vi "TL_convert_cluster into_TDMS_array.vi"(2 "TL cluster":T2={"405"=0.0, "488"=0.0, "561"=0.0, "641"=0.0, "BF "=0.0, "405 setpoint"=FALSE, "488 setpoint"=FALSE, "561 setpoint"=FALSE, "641 setpoint"=FALSE, "BF setpoint"=FALSE, "N planes 405"=0, "Dz 405"=0, "N planes 488"=0, "Dz 488"=0, "N planes 561"=0, "Dz 561"=0, "N planes 641"=0, "Dz 641"=0, "N planes BF"=0, "Dz BF"=0, "Tau 405"=inf, "Tau 488"=inf, "Tau 561"=inf, "Tau 641"=inf, "Tau BF"=inf, "405 set"=FALSE, "488 set "=FALSE, "561 set"=FALSE, "641 set"=FALSE, "BF set"=FALSE} {"Tau BF" format="%#_6e"; "Tau 641" format="%#_6e"; "Tau 561" format="%#_6e"; "Tau 488" format="%#_6e"; "Tau 405" format="%#_6e"; "641" min=0.0 max=100.0 step=0.1 scale=0.0..100.0; "561" min=0.0 max=100.0 step=0.1 scale=0.0..100.0; "405" min=0.0 max=100.0 step=0.1 scale=0.0..100.0; "488" min=0.0 max=100.0 step=0.1 scale=0.0..100.0; "BF" min=0.0 max=100.0 step=0.1 scale=0.0..100.0}, 3 "TL - setpoint cluster":T1) -> (0 "TL data for TDMS":cluster{dbl[][], dbl[][]})   [LabVIEW 2015]
uses:
  CONTROLS/Time_lapse_parameters.ctl
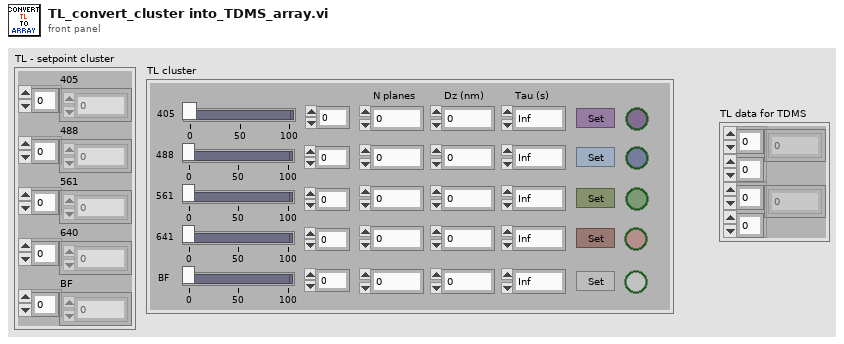
[diagram p1: front panel]
types:
  T1 = cluster{"405":dbl[], "488":dbl[], "561":dbl[], "640":dbl[], "BF":dbl[]}
  T2 = typedef "Time_lapse_parameters.ctl" = cluster{"405":dbl, "488":dbl, "561":dbl, "641":dbl, "BF ":dbl, "405 setpoint":bool, "488 setpoint":bool, "561 setpoint":bool, "641 setpoint":bool, "BF setpoint":bool, "N planes 405":i32, "Dz 405":i32, "N planes 488":i32, "Dz 488":i32, "N planes 561":i32, "Dz 561":i32, "N planes 641":i32, "Dz 641":i32, "N planes BF":i32, "Dz BF":i32, "Tau 405":dbl, "Tau 488":dbl, "Tau 561":dbl, "Tau 641":dbl, "Tau BF":dbl, "405 set":bool, "488 set ":bool, "561 set":bool, "641 set":bool, "BF set":bool}
  T3 = cluster{"Setpoint":dbl[][], "parameters":dbl[][]}
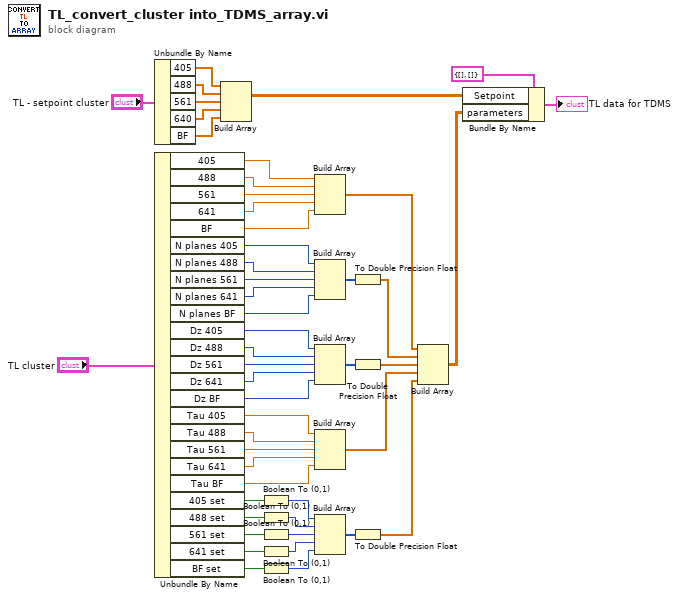
[diagram p0: block diagram]
diagram:
  n1 = Unbundle By Name("TL - setpoint cluster") -> ("405"=w9:dbl[], "488"=w8:dbl[], "561"=w7:dbl[], "640"=w6:dbl[], "BF"=w5:dbl[])
  n2 = Unbundle By Name("TL cluster") -> ("405"=w48:dbl, "488"=w47:dbl, "561"=w46:dbl, "641"=w45:dbl, "BF"=w44:dbl, "N planes 405"=w22:i32, "N planes 488"=w21:i32, "N planes 561"=w20:i32, "N planes 641"=w19:i32, "N planes BF"=w18:i32, "Dz 405"=w17:i32, "Dz 488"=w16:i32, "Dz 561"=w15:i32, "Dz 641"=w14:i32, "Dz BF"=w13:i32, "Tau 405"=w41:dbl, "Tau 488"=w42:dbl, "Tau 561"=w43:dbl, "Tau 641"=w40:dbl, "Tau BF"=w39:dbl, "405 set"=w38:bool, "488 set"=w37:bool, "561 set"=w36:bool, "641 set"=w35:bool, "BF set"=w34:bool)
  n3 = Build Array(w9, w8, w7, w6, w5) -> (w4:dbl[][])
  n4 = Boolean To (0,1)(Boolean=w38) -> (0, 1=w33:i16)
  n5 = Boolean To (0,1)(Boolean=w37) -> (0, 1=w32:i16)
  n6 = Boolean To (0,1)(Boolean=w36) -> (0, 1=w31:i16)
  n7 = Boolean To (0,1)(Boolean=w35) -> (0, 1=w30:i16)
  n8 = Boolean To (0,1)(Boolean=w34) -> (0, 1=w29:i16)
  n9 = Build Array(w48, w47, w46, w45, w44) -> (w28:dbl[])
  n10 = Build Array(w22, w21, w20, w19, w18) -> (w27:i32[])
  n11 = Build Array(w17, w16, w15, w14, w13) -> (w26:i32[])
  n12 = Build Array(w41, w42, w43, w40, w39) -> (w25:dbl[])
  n13 = Build Array(w33, w32, w31, w30, w29) -> (w24:i16[])
  n14 = To Double Precision Float(number=w27) -> (double precision float=w11:dbl[])
  n15 = To Double Precision Float(number=w26) -> (double precision float=w12:dbl[])
  n16 = To Double Precision Float(number=w24) -> (double precision float=w23:dbl[])
  n17 = Build Array(w28, w11, w12, w25, w23) -> (w1:dbl[][])
  n18 = Bundle By Name(cluster=T3 {"Setpoint"=[], "parameters"=[]} ("output cluster"), "Setpoint"=w4, "parameters"=w1) -> (→"TL data for TDMS":T3)
